vi "LaunchVI_BG.vi"(8 "error in":errorcluster, 11 "vi path":path) -> (0 "error out":errorcluster, 3 "reference out":refnum<vi>)   [LabVIEW 2011]
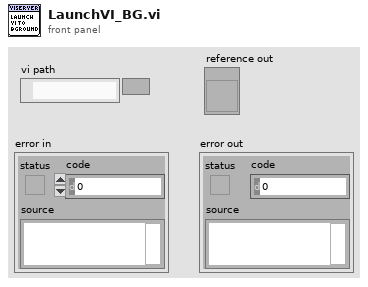
[diagram p1: front panel]
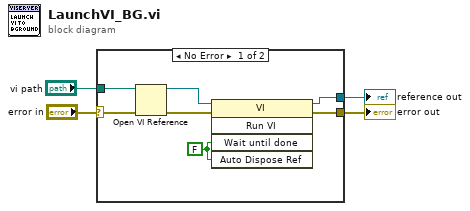
[diagram p0: block diagram]
diagram:
  n1 = case shown="No Error" "error in" {
    selector: "error in" -> [w5 w12]
    tunnel: [w11 w12] -> w4
    tunnel: "vi path" -> [w7 _]
    tunnel: [w6 _] -> w2
    frame No Error {
      w8 = FALSE ("Wait Until Done")
      n2 = Open VI Reference(vi path=w7, error in (no error)=w5) -> (vi reference=w10:refnum<vi>, error out=w9:errorcluster)  [unwired: 4 in]
      n3 = invoke class="VI" method="Run VI"(reference=w10, error in=w9, "Wait until done"=w8, "Auto Dispose Ref"=w8) -> (reference out=w6:refnum<vi>, error out=w11:errorcluster)  [unwired: 1 in, 3 out]
    }
    frame Error {
    }
  }
  "error out" <- w4
  "reference out" <- w2
